vi "Calc Power.vi"(1 "Value":sgl, 2 "Power":i32) -> (0 "Result":sgl)   [LabVIEW 2021]
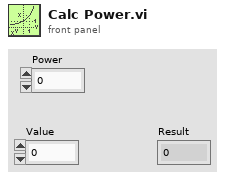
[diagram p1: front panel]
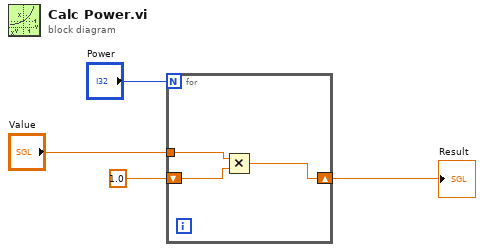
[diagram p0: block diagram]
diagram:
  n1 = for {
    N: "Power" -> [_]
    shift-right: [w5] -> w4
    shift-left: sgl 1.0 -> [w7]
    tunnel: "Value" -> [w6]
    n2 = Multiply(x=w6, y=w7) -> (x*y=w5:sgl)
  }
  "Result" <- w4
